vi "uTTA_ReadDirectory.vi"(8 "error in":errorcluster, 10 "Directory Name":string="/", 11 "VISA Refnum in":refnum<visa-resource-name>) -> (0 "error out":errorcluster, 2 "Files":string[](array[string]), 3 "VISA Refnum out":refnum<visa-resource-name>)   [LabVIEW 2021]
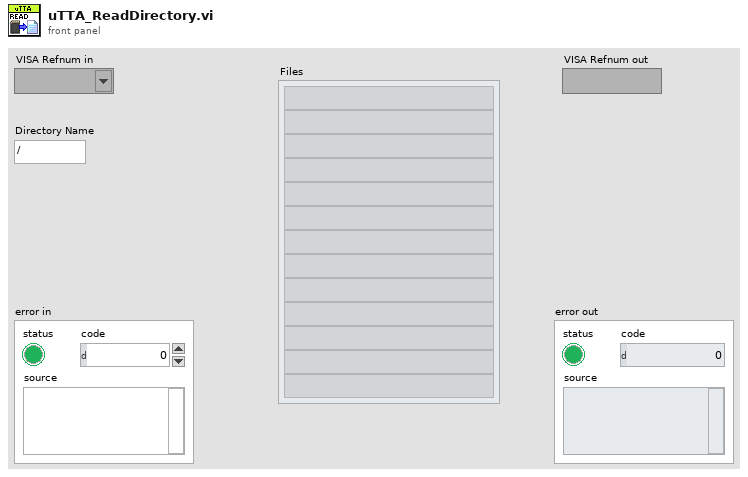
[diagram p1: front panel]
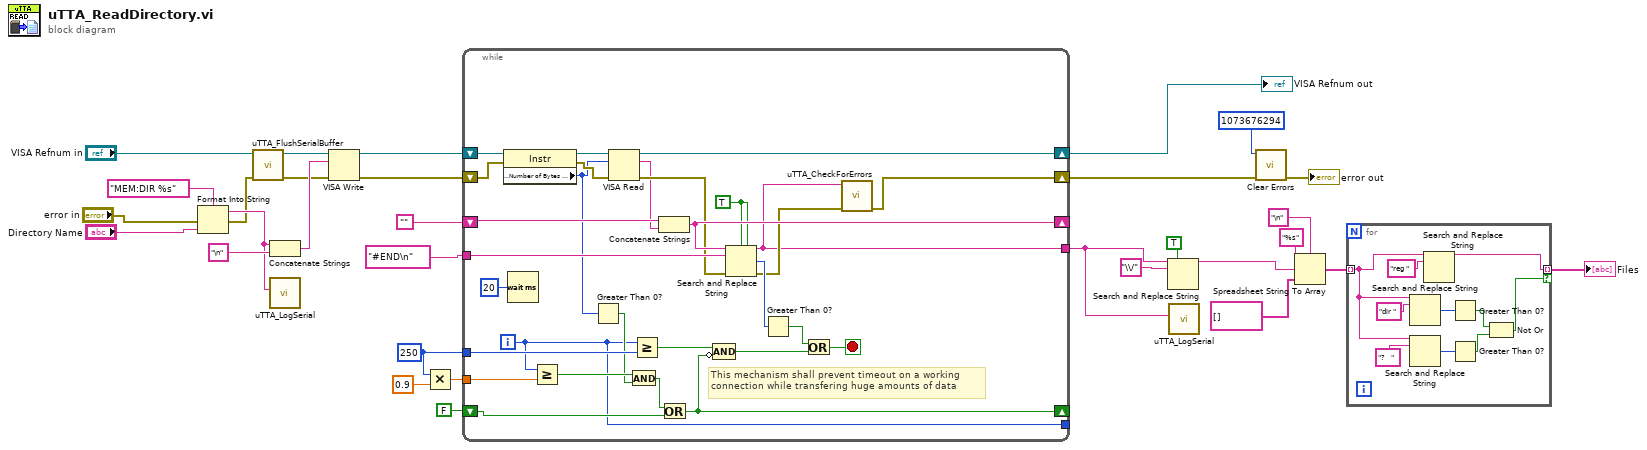
[diagram p0: block diagram]
diagram:
  w23 = 250 ("Timeout(ms)")
  n1 = Format Into String(format string="MEM:DIR %s", error in="error in", "Directory Name") -> (resulting string=w6:string, error out=w3:errorcluster)  [unwired: 1 in]
  n2 = call "uTTA_FlushSerialBuffer.vi"("error in (no error)"=w3, "VISA Refnum in"="VISA Refnum in") -> ("error out"=w2:errorcluster, "VISA Refnum out"=w1:refnum<visa-resource-name>)  [unwired: 4 in]
  n3 = Concatenate Strings(w6, "\n" ("delimiter (Tab)")) -> (w7:string)
  n4 = call "uTTA_LogSerial.vi"("Data_Sent"=w6) -> ()  [unwired: 6 in, 1 out]
  n5 = VISA Write(VISA resource name=w1, write buffer=w7, error in (no error)=w2) -> (VISA resource name out=w27:refnum<visa-resource-name>, error out=w28:errorcluster)  [unwired: 1 out]
  n6 = Multiply(x=w23, y=0.9) -> (x*y=w21:dbl)
  n7 = while {
    shift-right: [w55] -> _
    shift-left: "" -> [w56]
    tunnel: [w32] -> w5
    shift-right: [w46] -> w17
    shift-left: w28 -> [w59]
    shift-right: [w52] -> w24
    shift-left: w27 -> [w60]
    tunnel: w23 -> [w49]
    tunnel: "#END\n" ("RX Termination(\\n)") -> [w48]
    tunnel: w21 -> [w44]
    shift-right: [w38] -> _
    shift-left: FALSE ("ignore case? (F)") -> [w39]
    tunnel: [w35] -> _
    i -> [w35]
    stop <- w50 stop-if-true
    w45 = TRUE ("ignore case? (F)")
    # "This mechanism shall prevent timeout on a working\nconnection while transfering huge amounts of data"
    n8 = property class="Instr"(reference=w60, error in=w59) -> (reference out=w58:refnum<visa-resource-name>, error out=w57:errorcluster, "Serial Settings:Number of Bytes at Serial Port"=w42:u32)
    n9 = Wait (ms)(milliseconds to wait=u32 20) -> ()  [unwired: 1 out]
    n10 = Greater Or Equal?(x=w35, y=w44) -> (x >= y?=w43:bool)
    n11 = Greater Than 0?(x=w42) -> (x > 0?=w41:bool)
    n12 = VISA Read(VISA resource name=w58, byte count=w42, error in (no error)=w57) -> (VISA resource name out=w52:refnum<visa-resource-name>, read buffer=w33:string, error out=w34:errorcluster)  [unwired: 1 out]
    n13 = And(x=w43, y=w41) -> (x .and. y?=w40:bool)
    n14 = Greater Or Equal?(x=w35, y=w49) -> (x >= y?=w37:bool)
    n15 = Concatenate Strings(w56, w33) -> (w55:string)
    n16 = Or(x=w40, y=w39) -> (x .or. y?=w38:bool)
    n17 = Compound Arithmetic op=AND(w37, invert w38) -> (w36:bool)
    n18 = Search and Replace String(case sensitive?=w45, multiline?=w45, input string=w55, search string=w48, error in=w34) -> (result string=w32:string, number of replacements=w54:i32, error out=w47:errorcluster)  [unwired: 3 in, 1 out]
    n19 = Greater Than 0?(x=w54) -> (x > 0?=w51:bool)
    n20 = Or(x=w51, y=w36) -> (x .or. y?=w50:bool)
    n21 = call "uTTA_CheckForErrors.vi"("error in"=w47, "Received"=w32) -> ("error out"=w46:errorcluster)  [unwired: 9 in]
  }
  "VISA Refnum out" <- w24
  n22 = Search and Replace String(replace all?=TRUE ("replace all? (F)"), input string=w5, search string="\\/") -> (result string=w13:string)  [unwired: 5 in, 3 out]
  n23 = call "uTTA_LogSerial.vi"("Data_Sent"=w5) -> ()  [unwired: 6 in, 1 out]
  n24 = call <vilib>:"Clear Errors.vi"("error in (no error)"=w17, "specific error code to clear (0: all)"=1073676294) -> ("error out"=→"error out":errorcluster)  [unwired: 4 in, 1 out]
  n25 = Spreadsheet String To Array(delimiter (Tab)="\n", format string="%s", spreadsheet string=w13, array type (2D Dbl)=string[] []) -> (array=w10:string[])
  n26 = for {
    tunnel: w10 -> [w62] mode=indexing
    tunnel: [w61] -> w9 mode=indexing if=w64
    n27 = Search and Replace String(input string=w62, search string="dir ") -> (number of replacements=w68:i32)  [unwired: 6 in, 3 out]
    n28 = Search and Replace String(input string=w62, search string="?   ") -> (number of replacements=w67:i32)  [unwired: 6 in, 3 out]
    n29 = Search and Replace String(input string=w62, search string="reg ") -> (result string=w61:string)  [unwired: 6 in, 3 out]
    n30 = Greater Than 0?(x=w68) -> (x > 0?=w66:bool)
    n31 = Greater Than 0?(x=w67) -> (x > 0?=w65:bool)
    n32 = Not Or(1:w65, 2:w66) -> (0:w64:bool)
  }
  "Files" <- w9
